vi "Core-Engine.vi"(7 "Ctrl-Refs":T1, 8 "Err-I":errorcluster, 9 "ErrQRef":refnum<queue>, 11 "MainQ-I":refnum<queue>) -> (0 "Err-O":errorcluster)   [LabVIEW 2020]
doc: "Main State Machine LOOP of Core.\nThis vi act as an engine to pump application run."
uses:
  Core-CtrlRefs.ctl
panel:
  # "Outputs"
  # "Inputs"
  # ":: Modularized Parallism Templete ::\n- Main State Machine -\nby: Gaoke Yang <gaoke.yang@yahoo.com>\nhttp://www.mViAcademy.com\nCopyright (C) 2010, mVi Academy All Rights Reserved"
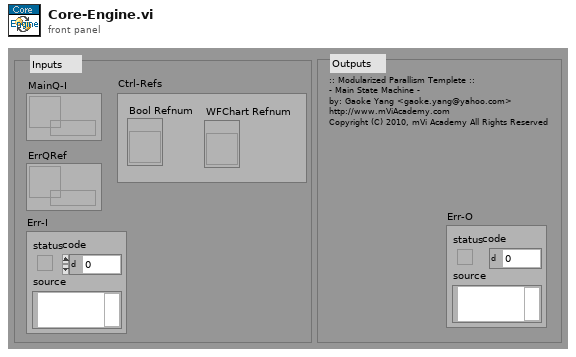
[diagram p1: front panel]
types:
  T1 = typedef "Core-CtrlRefs.ctl" = cluster{"Bool Refnum":refnum<vi>, "WFChart Refnum":refnum<vi>}
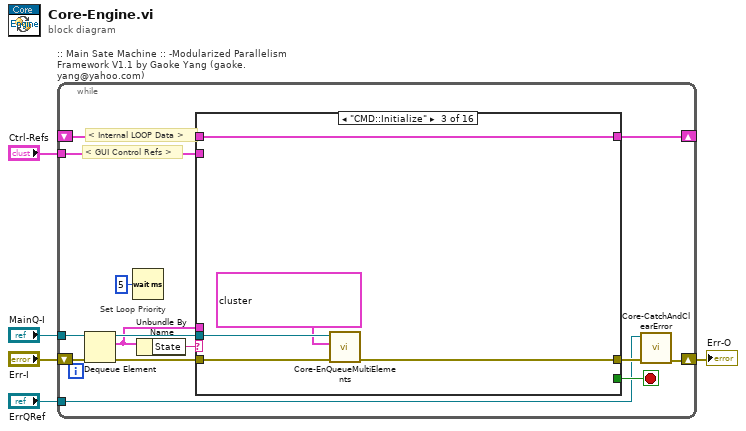
[diagram p0: block diagram]
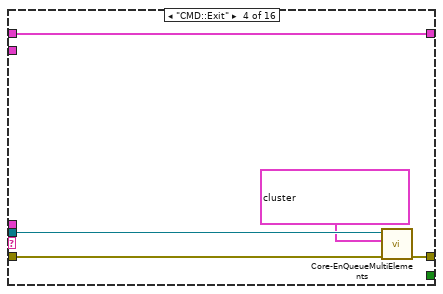
[diagram p4: hidden frame]
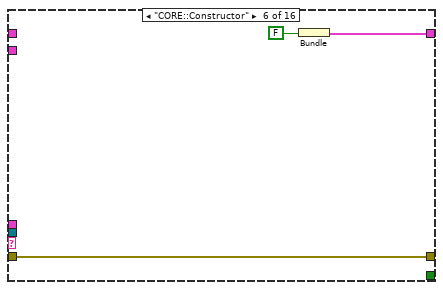
[diagram p6: hidden frame]
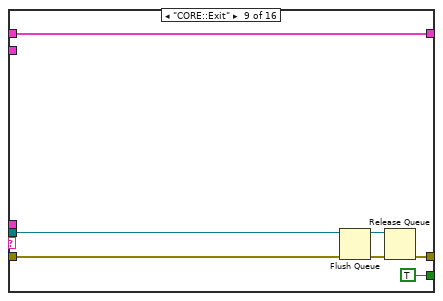
[diagram p9: hidden frame]
diagram:
  n1 = while ":: Main Sate Machine :: -Modularized Parallelism Framework V1.1 by Gaoke Yang (gaoke.yang@yahoo.com)" {
    tunnel: "MainQ-I" -> [w19]
    shift-right: [w8] -> w2
    shift-left: "Err-I" -> [w10]
    shift-right: [w13] -> _
    shift-left: _ -> [w12]
    tunnel: "Ctrl-Refs" -> [w11]
    tunnel: "ErrQRef" -> [w7]
    stop <- w16 stop-if-true
    # "Set Loop Priority"
    # "< GUI Control Refs >"
    # "< Internal LOOP Data >"
    n2 = Dequeue Element(queue=w19, error in (no error)=w10) -> (queue out=w17:refnum<queue>, element=w14:cluster{"State":string, "Data":variant}, error out=w18:errorcluster)  [unwired: 2 out]
    n3 = Wait (ms)(milliseconds to wait=u32 5) -> ()  [unwired: 1 out]
    n4 = Unbundle By Name(w14) -> ("State"=w15:string)
    n5 = case shown="\"CMD::Initialize\"" w15 {
      tunnel: [w20 w23 w27 w32 w35 w38 w40 w42 w45 w50 w52 w54 w57 w59 w61 w62] -> w9
      tunnel: [_ _ _ _ _ _ _ _ TRUE _ _ _ _ _ _ _] -> w16
      tunnel: w17 -> [_ _ w28 w31 _ _ _ _ w48 _ _ _ _ _ _ _]
      tunnel: w18 -> [w20 w23 w24 w33 w35 w38 w40 w42 w47 w50 w52 w54 w57 w59 w61 w62]
      tunnel: w14 -> [_ _ _ _ _ _ _ _ _ _ _ _ _ _ _ _]
      tunnel: [w21 w22 w25 w29 w34 w36 w39 w41 w43 w51 w53 w55 w56 w58 w60 w63] -> w13
      tunnel: w12 -> [w21 w22 w25 w29 w34 _ w39 w41 w43 w51 w53 w55 w56 w58 w60 w63]
      tunnel: w11 -> [_ _ _ _ _ _ _ _ _ _ _ _ _ _ _ _]
      frame "IDLE", Default {
      }
      frame "-------- Commands ---------" {
      }
      frame "CMD::Initialize" {
        n6 = call "Core-EnQueueMultiElements.vi"("ErrorIn"=w24, "CmdArray"=cluster{"State":string, "Data":variant}[] [{"State"="CORE::Constructor", "Data"=variant}, {"State"="CORE::Initialize", "Data"=variant}], "QRefIn"=w28) -> ("ErrorOut"=w27:errorcluster)  [unwired: 8 in]
      }
      frame "CMD::Exit" {
        n7 = call "Core-EnQueueMultiElements.vi"("ErrorIn"=w33, "CmdArray"=cluster{"State":string, "Data":variant}[] [{"State"="CORE::DeConstructor", "Data"=variant}, {"State"="CORE::Exit", "Data"=variant}], "QRefIn"=w31) -> ("ErrorOut"=w32:errorcluster)  [unwired: 8 in]
      }
      frame "------------ Core ------------" {
      }
      frame "CORE::Constructor" {
        n8 = Bundle(FALSE) -> (w36:cluster{bool})  [unwired: 1 in]
      }
      frame "CORE::Initialize" {
      }
      frame "CORE::DeConstructor" {
      }
      frame "CORE::Exit" {
        n9 = Flush Queue(queue=w48, error in (no error)=w47) -> (queue out=w44:refnum<queue>, error out=w46:errorcluster)  [unwired: 1 out]
        n10 = Release Queue(queue=w44, error in (no error)=w46) -> (error out=w45:errorcluster)  [unwired: 1 in, 2 out]
      }
      frame "------------  GUI  -------------" {
      }
      frame "GUI::Initialize" {
      }
      frame "GUI::SetCusor" {
      }
      frame "GUI::SetMenu" {
      }
      frame "----------- USER -----------" {
      }
      frame "USER::Case1" {
      }
      frame "USER::Case2" {
      }
    }
    n11 = call "Core-CatchAndClearError.vi"("Err-I"=w9, "ErrQ-I"=w7) -> ("Err-O"=w8:errorcluster)  [unwired: 9 in]
  }
  "Err-O" <- w2
